vi "Write Plot Names.vi"(8 "error in (no error)":errorcluster, 10 "Names":string[](array[string]), 11 "Graph in":refnum<vi>) -> (0 "error out":errorcluster, 3 "Graph":refnum<vi>)   [LabVIEW 2020, in "VolatusGUIEditorCore.lvlib"]
uses:
  VolatusGUIEditorCore.lvlib
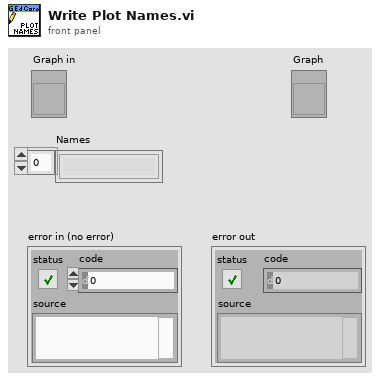
[diagram p1: front panel]
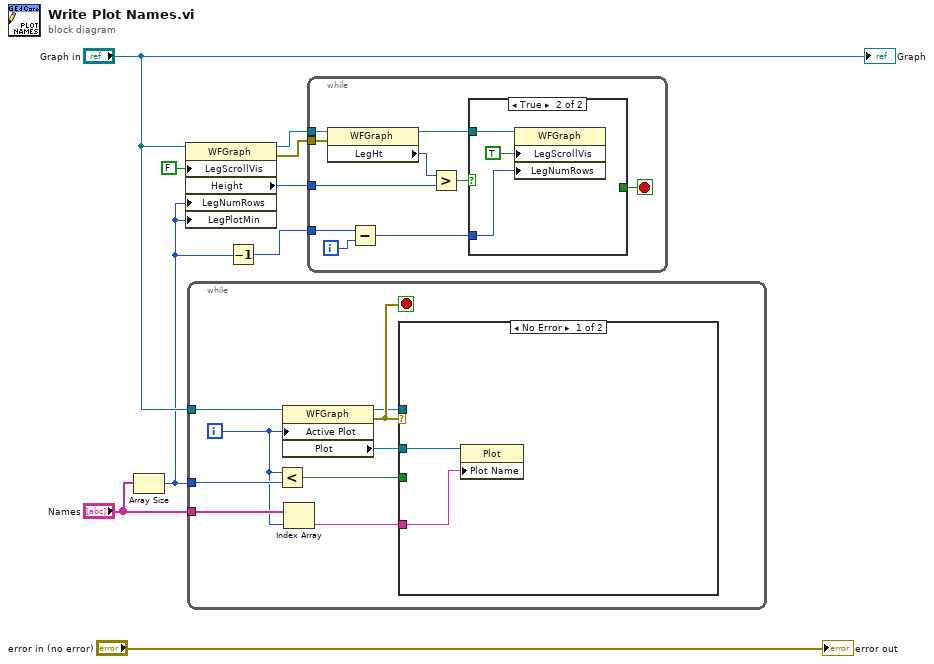
[diagram p0: block diagram]
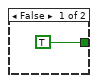
[diagram p2: hidden frame]
diagram:
  n1 = Array Size(array="Names") -> (size(s)=w1:i32)
  n2 = property class="WFGraph"(reference="Graph in", "LegScrollVis"=FALSE ("Legend:Scrollbar Visible"), "LegNumRows"=w1, "LegPlotMin"=w1) -> (reference out=w6:refnum<vi>, error out=w5:errorcluster, "Height"=w4:u32)  [unwired: 1 in]
  n3 = while {
    tunnel: "Graph in" -> [w16]
    tunnel: "Names" -> [w12]
    tunnel: w1 -> [w17]
    i -> [w11]
    stop <- w18 stop-if-true
    n4 = Less?(x=w11, y=w17) -> (x < y?=w13:bool)
    n5 = property class="WFGraph"(reference=w16, "Active Plot"=w11) -> (reference out=w15:refnum<vi>, error out=w18:errorcluster, "Plot"=w14:refnum<vi>)  [unwired: 1 in]
    n6 = Index Array(array=w12, index=w11) -> (element=w10:string)
    n7 = case shown="No Error" w18 {
      tunnel: w15 -> [_ _]
      tunnel: w14 -> [w19 _]
      tunnel: w13 -> [_ _]
      tunnel: w10 -> [w20 _]
      frame No Error {
        n8 = property class="Plot"(reference=w19, "Plot Name"=w20) -> ()  [unwired: 1 in, 2 out]
      }
      frame Error {
      }
    }
  }
  n9 = Decrement(x=w1) -> (x-1=w3:i32)
  n10 = while {
    tunnel: w6 -> [w30]
    tunnel: w5 -> [w29]
    tunnel: w4 -> [w28]
    tunnel: w3 -> [w26]
    i -> [w25]
    stop <- w21 stop-if-true
    n11 = property class="WFGraph"(reference=w30, error in=w29) -> (reference out=w22:refnum<vi>, "LegHt"=w27:u32)  [unwired: 1 out]
    n12 = Subtract(x=w26, y=w25) -> (x-y=w24:i32)
    n13 = Greater?(x=w27, y=w28) -> (0:w23:bool)
    n14 = case shown="True" w23 {
      tunnel: w24 -> [_ w33]
      tunnel: w22 -> [_ w34]
      tunnel: [TRUE _] -> w21
      frame False {
      }
      frame True {
        n15 = property class="WFGraph"(reference=w34, "LegScrollVis"=TRUE ("Legend:Scrollbar Visible"), "LegNumRows"=w33) -> ()  [unwired: 1 in, 2 out]
      }
    }
  }
  "Graph" <- "Graph in"
  "error out" <- "error in (no error)"
